vi "CThread Activate Killswitch.vi"(8 "2nd Button (Optional)":T3(ring), 9 "1st Button":T3(ring), 10 "Mode (1st Button Only)":T2(ring), 11 "NXT":T1) -> (3 "NXT":T1)   [LabVIEW 2010, in "FTC.lvlib"]
uses:
  FTC.lvlib
  <vilib>/NXT/Subs/LVHSConnector.ctl
  CLIB/CThread/Core/CThread Thread Properties.ctl
  CLIB/CRef/Interface/CRef Boolean.llb/Boolean CReference.ctl
  CLIB/CThread/XNodes/referencenode/CThread VI Reference.xnode
  CLIB/CThread/XNodes/terminalnode/CThread VI Terminal Node.xnode
  CLIB/CThread/Base/CThread Base - VI Reference.vi
  CLIB/CThread/Base/CThread Base - While Loop.vi
  CLIB/CThread/CThread.lvlib
  CLIB/CRef/CRef.lvlib
  CLIB/CRef/Interface/CRef Numeric.llb/I32 CReference.ctl
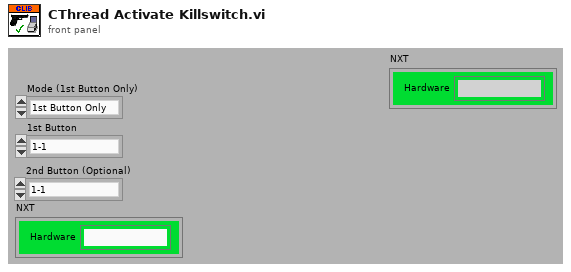
[diagram p1: front panel]
types:
  T1 = typedef "LVHSConnector.ctl" = cluster{"Hardware":string, "Flattened String":string}
  T2 = enum16{"1st Button Only", "1st AND 2nd Buttons", "1st OR 2nd Button"}
  T3 = enum16{"1-1", "1-2", "1-3", "1-4", "1-5", "1-6", "1-7", "1-8", "1-9", "1-10", "1-11", "1-12", "2-1", "2-2", "2-3", "2-4", "2-5", "2-6", "2-7", "2-8", "2-9", "2-10", "2-11", "2-12", "NXT-L", "NXT-R", "NXT-E", "1-U", "1-UR", "1-R", "1-DR", "1-D", "1-DL", "1-L", "1-UL", "2-U", "2-UR", "2-R", "2-DR", "2-D", "2-DL", "2-L", "2-UL"}
  T4 = typedef "CThread.lvlib/CThread Thread Properties.ctl" = cluster{"Post-Run Delay (5ms)":u32}
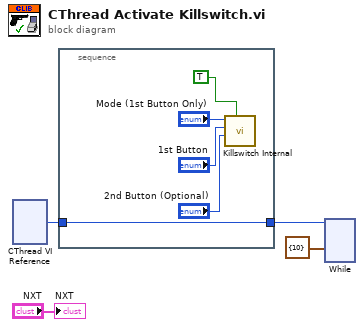
[diagram p0: block diagram]
diagram:
  n1 = xnode "CThread VI Reference"() -> ("Killswitch Internal.vi"=w4:i32)
  n2 = stacked-sequence {
    tunnel: w4 -> [w5]
    tunnel: [w5] -> w1
    frame #0 {
      n3 = call "Killswitch Internal.vi"("Writing? (F)"=TRUE, "Write 2nd Button"="2nd Button (Optional)", "Write 1st Button"="1st Button", "Write Mode"="Mode (1st Button Only)") -> ()  [unwired: 8 in]
    }
  }
  n4 = xnode "While"("CLIB VI Reference"=w1, "Thread Properties"=T4 {"Post-Run Delay (5ms)"=10}) -> ()  [unwired: 1 in, 2 out]
  "NXT" <- "NXT"
